vi "CheckSum Append.vi"(8 "error in (no error)":errorcluster, 10 "Input Cmd":string) -> (0 "error out":errorcluster, 2 "ChkSum Cmd":string)   [LabVIEW 2012, in "TDK-Lambda Z.lvlib"]
doc: "This VI will add a checksum to any command string.\nThe format of the \"ChkSum Cmd\" output is:\n \"Command\" & \"Dollar Sign\" & \"Two Hex Digits\" & \"Carriage Return\"\n\nThe command is only formulated, it is not sent to the instrument.\n\nAppend \"$xx\" checksum to any command string if it is not already done"
uses:
  TDK-Lambda Z.lvlib
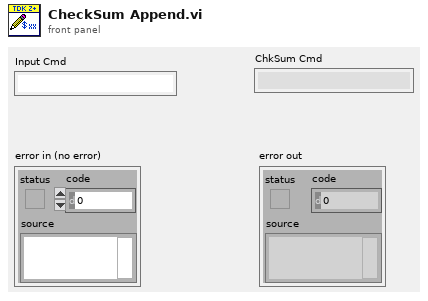
[diagram p1: front panel]
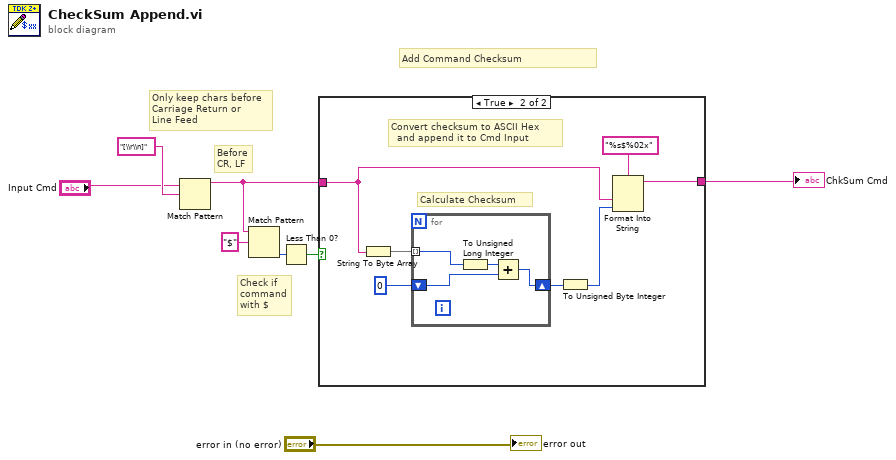
[diagram p0: block diagram]
diagram:
  # "Check if \ncommand\nwith $"
  # "Add Command Checksum"
  # "Before\nCR, LF"
  # "Only keep chars before\nCarriage Return or\nLine Feed"
  n1 = Match Pattern(string="Input Cmd", regular expression="[\\r\\n]") -> (before substring=w4:string)  [unwired: 1 in, 3 out]
  n2 = Match Pattern(string=w4, regular expression="$") -> (offset past match=w3:i32)  [unwired: 1 in, 3 out]
  n3 = Less Than 0?(x=w3) -> (x < 0?=w2:bool)
  n4 = case shown="True" w2 {
    tunnel: w4 -> [w9 w16]
    tunnel: [w9 w10] -> w6
    frame False {
      # "command\nwith $"
    }
    frame True {
      # "Convert checksum to ASCII Hex  \n  and append it to Cmd Input"
      # "Calculate Checksum"
      n5 = String To Byte Array(string=w16) -> (unsigned byte array=w15:u8[])
      n6 = for {
        tunnel: w15 -> [w20] mode=indexing
        shift-right: [w18] -> w13
        shift-left: u32 0 -> [w19]
        n7 = To Unsigned Long Integer(number=w20) -> (unsigned 32bit integer=w17:u32)
        n8 = Add(x=w17, y=w19) -> (x+y=w18:u32)
      }
      n9 = To Unsigned Byte Integer(number=w13) -> (unsigned 8bit integer=w11:u8)
      n10 = Format Into String(format string="%s$%02x" ("regular expression"), w16, w11) -> (resulting string=w10:string)  [unwired: 2 in, 1 out]
    }
  }
  "ChkSum Cmd" <- w6
  "error out" <- "error in (no error)"
